vi "Configure Position Offset.vi"(8 "error in (no error)":errorcluster, 10 "CCW Position Offset (0.0 rad)":dbl, 11 "Hitec HS400 Series FPGA in":refnum<class "Hitec HS400 Series FPGA.lvclass">) -> (0 "error out":errorcluster, 3 "Hitec HS400 Series FPGA out":refnum<class "Hitec HS400 Series FPGA.lvclass">)   [LabVIEW 2013, in "Hitec HS400 Series FPGA.lvclass"]
doc: "Configures the counterclockwise software position offset."
uses:
  Hitec HS400 Series FPGA.lvclass
  Hitec HS400 Series FPGA.lvclass/Hitec HS400 Series FPGA.ctl
  <vilib>/rvi/interface/common/niFpgaWaitOnOcc.vi
  <vilib>/rvi/errors/niLvFpgaAdjustHostInterfaceError.vi
  <vilib>/rvi/interface/nirviReadWriteControl/nirviReadWriteControl.xnode
  NiFpgaLv.dll
  <vilib>/rvi/interface/Simulation/niFpgaSimulationCallBeginRW.vi
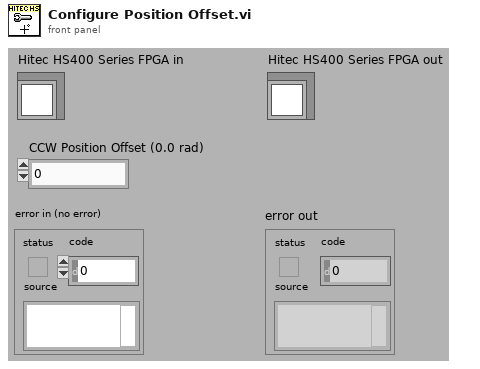
[diagram p1: front panel]
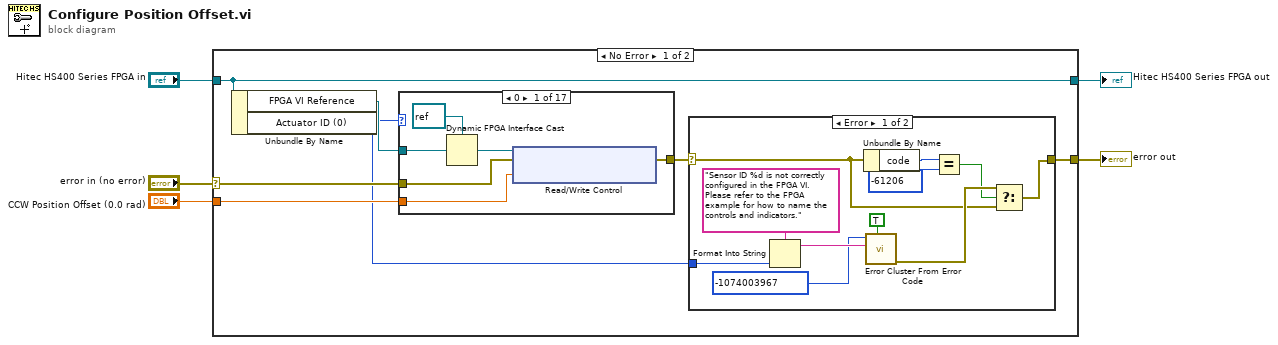
[diagram p0: block diagram]
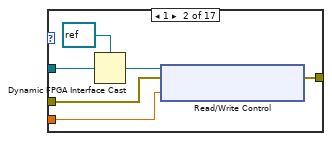
[diagram p3: hidden frame]
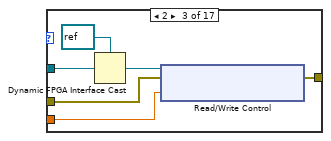
[diagram p4: hidden frame]
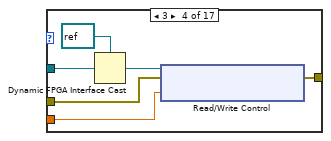
[diagram p5: hidden frame]
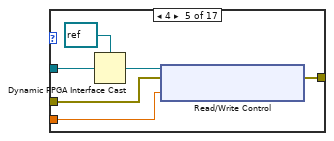
[diagram p6: hidden frame]
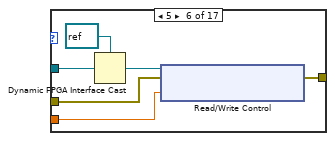
[diagram p7: hidden frame]
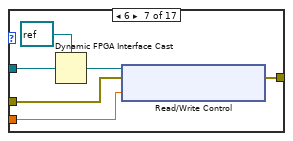
[diagram p8: hidden frame]
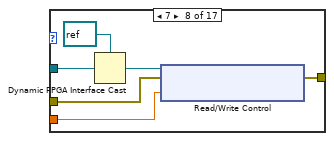
[diagram p9: hidden frame]
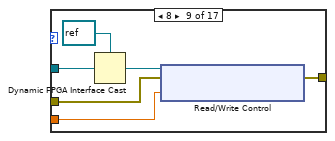
[diagram p10: hidden frame]
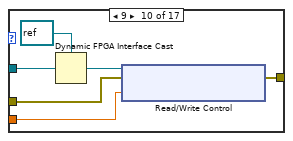
[diagram p11: hidden frame]
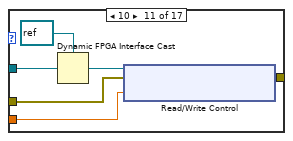
[diagram p12: hidden frame]
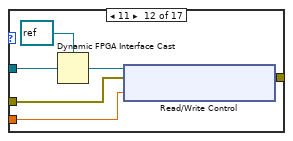
[diagram p13: hidden frame]
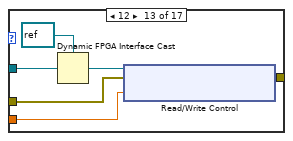
[diagram p14: hidden frame]
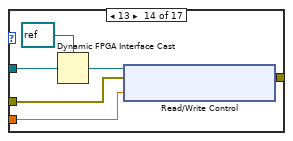
[diagram p15: hidden frame]
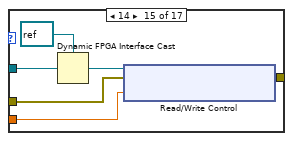
[diagram p16: hidden frame]
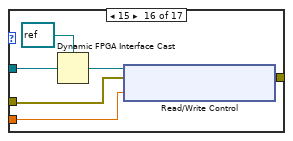
[diagram p17: hidden frame]
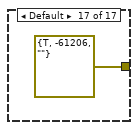
[diagram p18: hidden frame]
diagram:
  n1 = case shown="No Error" "error in (no error)" {
    selector: "error in (no error)" -> [w12 w123]
    tunnel: [w6 w123] -> w2
    tunnel: [w11 w122] -> w3
    tunnel: "Hitec HS400 Series FPGA in" -> [w11 w122]
    tunnel: "CCW Position Offset (0.0 rad)" -> [w9 _]
    frame No Error {
      n2 = Unbundle By Name(w11) -> ("FPGA VI Reference"=w10:refnum<k20>, "Actuator ID (0)"=w7:i32)
      n3 = case shown="0" w7 {
        tunnel: w10 -> [w30 w35 w41 w47 w53 w59 w65 w71 w77 w83 w89 w95 w101 w107 w113 w119 _]
        tunnel: w12 -> [w28 w34 w40 w46 w52 w58 w64 w70 w76 w81 w88 w93 w99 w105 w112 w118 _]
        tunnel: [w27 w33 w39 w45 w51 w57 w63 w69 w75 w82 w87 w94 w100 w106 w111 w117 errorcluster {"status"=TRUE, "code"=-61206, "source"=""} ("error out")] -> w8
        tunnel: w9 -> [w26 w32 w38 w44 w50 w56 w62 w68 w74 w80 w86 w92 w98 w104 w110 w116 _]
        frame 0 {
          n4 = Dynamic FPGA Interface Cast(Session In=refnum<k20> refnum ("FPGA VI Reference Out"), Type=w30) -> (Session Out=w29:refnum<k20>)
          n5 = xnode "Read/Write Control"("FPGA VI Reference In"=w29, "error in"=w28, "hs400_0_ccw offset"=w26) -> ("error out"=w27:errorcluster)  [unwired: 1 out]
        }
        frame 1 {
          n6 = Dynamic FPGA Interface Cast(Session In=refnum<k20> refnum ("FPGA VI Reference Out"), Type=w35) -> (Session Out=w36:refnum<k20>)
          n7 = xnode "Read/Write Control"("FPGA VI Reference In"=w36, "error in"=w34, "hs400_1_ccw offset"=w32) -> ("error out"=w33:errorcluster)  [unwired: 1 out]
        }
        frame 2 {
          n8 = Dynamic FPGA Interface Cast(Session In=refnum<k20> refnum ("FPGA VI Reference Out"), Type=w41) -> (Session Out=w42:refnum<k20>)
          n9 = xnode "Read/Write Control"("FPGA VI Reference In"=w42, "error in"=w40, "hs400_2_ccw offset"=w38) -> ("error out"=w39:errorcluster)  [unwired: 1 out]
        }
        frame 3 {
          n10 = Dynamic FPGA Interface Cast(Session In=refnum<k20> refnum ("FPGA VI Reference Out"), Type=w47) -> (Session Out=w48:refnum<k20>)
          n11 = xnode "Read/Write Control"("FPGA VI Reference In"=w48, "error in"=w46, "hs400_3_ccw offset"=w44) -> ("error out"=w45:errorcluster)  [unwired: 1 out]
        }
        frame 4 {
          n12 = Dynamic FPGA Interface Cast(Session In=refnum<k20> refnum ("FPGA VI Reference Out"), Type=w53) -> (Session Out=w54:refnum<k20>)
          n13 = xnode "Read/Write Control"("FPGA VI Reference In"=w54, "error in"=w52, "hs400_4_ccw offset"=w50) -> ("error out"=w51:errorcluster)  [unwired: 1 out]
        }
        frame 5 {
          n14 = Dynamic FPGA Interface Cast(Session In=refnum<k20> refnum ("FPGA VI Reference Out"), Type=w59) -> (Session Out=w60:refnum<k20>)
          n15 = xnode "Read/Write Control"("FPGA VI Reference In"=w60, "error in"=w58, "hs400_5_ccw offset"=w56) -> ("error out"=w57:errorcluster)  [unwired: 1 out]
        }
        frame 6 {
          n16 = Dynamic FPGA Interface Cast(Session In=refnum<k20> refnum ("FPGA VI Reference Out"), Type=w65) -> (Session Out=w66:refnum<k20>)
          n17 = xnode "Read/Write Control"("FPGA VI Reference In"=w66, "error in"=w64, "hs400_6_ccw offset"=w62) -> ("error out"=w63:errorcluster)  [unwired: 1 out]
        }
        frame 7 {
          n18 = Dynamic FPGA Interface Cast(Session In=refnum<k20> refnum ("FPGA VI Reference Out"), Type=w71) -> (Session Out=w72:refnum<k20>)
          n19 = xnode "Read/Write Control"("FPGA VI Reference In"=w72, "error in"=w70, "hs400_7_ccw offset"=w68) -> ("error out"=w69:errorcluster)  [unwired: 1 out]
        }
        frame 8 {
          n20 = Dynamic FPGA Interface Cast(Session In=refnum<k20> refnum ("FPGA VI Reference Out"), Type=w77) -> (Session Out=w78:refnum<k20>)
          n21 = xnode "Read/Write Control"("FPGA VI Reference In"=w78, "error in"=w76, "hs400_8_ccw offset"=w74) -> ("error out"=w75:errorcluster)  [unwired: 1 out]
        }
        frame 9 {
          n22 = Dynamic FPGA Interface Cast(Session In=refnum<k20> refnum ("FPGA VI Reference Out"), Type=w83) -> (Session Out=w84:refnum<k20>)
          n23 = xnode "Read/Write Control"("FPGA VI Reference In"=w84, "error in"=w81, "hs400_9_ccw offset"=w80) -> ("error out"=w82:errorcluster)  [unwired: 1 out]
        }
        frame 10 {
          n24 = Dynamic FPGA Interface Cast(Session In=refnum<k20> refnum ("FPGA VI Reference Out"), Type=w89) -> (Session Out=w90:refnum<k20>)
          n25 = xnode "Read/Write Control"("FPGA VI Reference In"=w90, "error in"=w88, "hs400_10_ccw offset"=w86) -> ("error out"=w87:errorcluster)  [unwired: 1 out]
        }
        frame 11 {
          n26 = Dynamic FPGA Interface Cast(Session In=refnum<k20> refnum ("FPGA VI Reference Out"), Type=w95) -> (Session Out=w96:refnum<k20>)
          n27 = xnode "Read/Write Control"("FPGA VI Reference In"=w96, "error in"=w93, "hs400_11_ccw offset"=w92) -> ("error out"=w94:errorcluster)  [unwired: 1 out]
        }
        frame 12 {
          n28 = Dynamic FPGA Interface Cast(Session In=refnum<k20> refnum ("FPGA VI Reference Out"), Type=w101) -> (Session Out=w102:refnum<k20>)
          n29 = xnode "Read/Write Control"("FPGA VI Reference In"=w102, "error in"=w99, "hs400_12_ccw offset"=w98) -> ("error out"=w100:errorcluster)  [unwired: 1 out]
        }
        frame 13 {
          n30 = Dynamic FPGA Interface Cast(Session In=refnum<k20> refnum ("FPGA VI Reference Out"), Type=w107) -> (Session Out=w108:refnum<k20>)
          n31 = xnode "Read/Write Control"("FPGA VI Reference In"=w108, "error in"=w105, "hs400_13_ccw offset"=w104) -> ("error out"=w106:errorcluster)  [unwired: 1 out]
        }
        frame 14 {
          n32 = Dynamic FPGA Interface Cast(Session In=refnum<k20> refnum ("FPGA VI Reference Out"), Type=w113) -> (Session Out=w114:refnum<k20>)
          n33 = xnode "Read/Write Control"("FPGA VI Reference In"=w114, "error in"=w112, "hs400_14_ccw offset"=w110) -> ("error out"=w111:errorcluster)  [unwired: 1 out]
        }
        frame 15 {
          n34 = Dynamic FPGA Interface Cast(Session In=refnum<k20> refnum ("FPGA VI Reference Out"), Type=w119) -> (Session Out=w120:refnum<k20>)
          n35 = xnode "Read/Write Control"("FPGA VI Reference In"=w120, "error in"=w118, "hs400_15_ccw offset"=w116) -> ("error out"=w117:errorcluster)  [unwired: 1 out]
        }
        frame Default {
        }
      }
      n36 = case shown="Error" w8 {
        selector: w8 -> [w13 w24]
        tunnel: w7 -> [w16 _]
        tunnel: [w15 w24] -> w6
        frame Error {
          n37 = Format Into String(format string="Sensor ID %d is not correctly configured in the FPGA VI. Please refer to the FPGA example for how to name the controls and indicators." ("Source (VI Name)"), w16) -> (resulting string=w20:string)  [unwired: 2 in, 1 out]
          n38 = Unbundle By Name(w13) -> ("code"=w21:i32)
          n39 = call <vilib>:"Error Cluster From Error Code.vi"("show call chain? (False)"=TRUE, "error message (\"\")"=w20, "error code (0)"=-1074003967 ("Code")) -> ("error out"=w23:errorcluster)  [unwired: 6 in]
          n40 = Equal?(x=w21, y=-61206) -> (x = y?=w22:bool)
          n41 = Select(t=w23, s=w22, f=w13) -> (s? t:f=w15:errorcluster)
        }
        frame No Error {
        }
      }
    }
    frame Error {
    }
  }
  "error out" <- w2
  "Hitec HS400 Series FPGA out" <- w3
